vi "控件属性对话框.vi"() -> ()   [LabVIEW 2013]
panel:
  in  "选项卡控件":enum32{"外观", "数据类型", "数据输入", "显示格式"}(tab)
  in  "字符串":string
  in  "可见":bool
  # "标签"
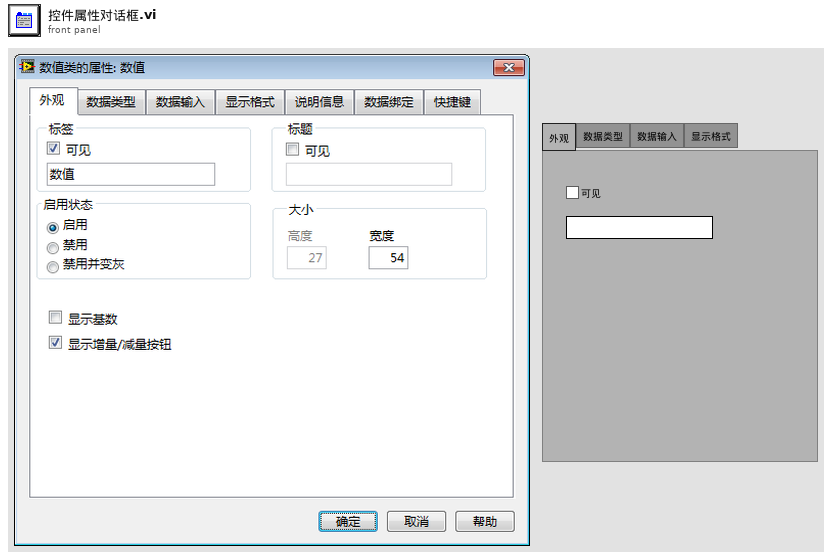
[diagram p1: front panel]
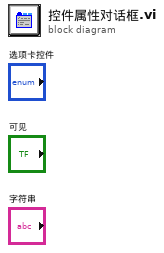
[diagram p0: block diagram]
diagram:
